vi "SaveImagesFromArray (SubVI).vi"(8 "error in (no error)":errorcluster, 9 "Array of Images":T1[](array[typedef]), 10 "XY Camera Coordinates":dbl[][](array[numeric]), 11 "Path to save collected images":path=path "E:/XYZstage+Camera_CollectedImages/12-17-2016/images") -> (0 "error out":errorcluster)   [LabVIEW 2016]
uses:
  <vilib>/vision/Image Controls.llb/IMAQ Image.ctl
  <vilib>/Utility/file.llb/Write Delimited Spreadsheet (DBL).vi
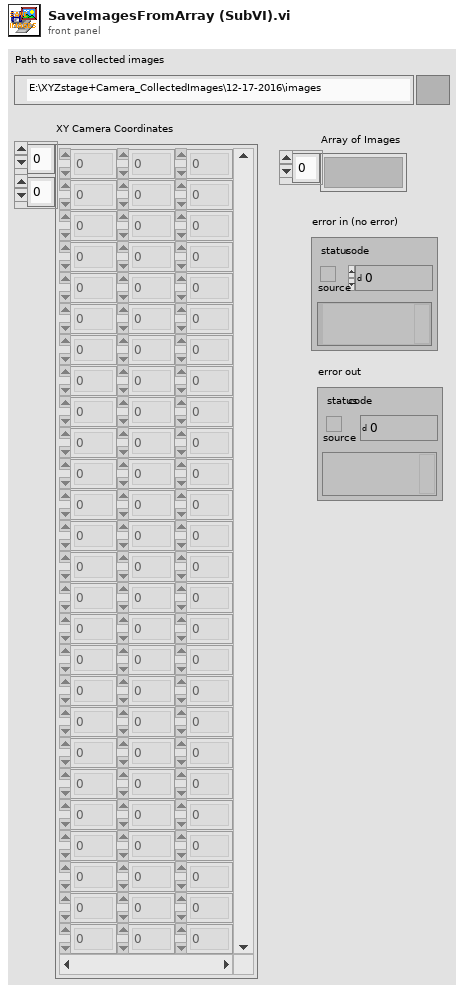
[diagram p1: front panel]
types:
  T1 = typedef "IMAQ Image.ctl" = refnum<image>
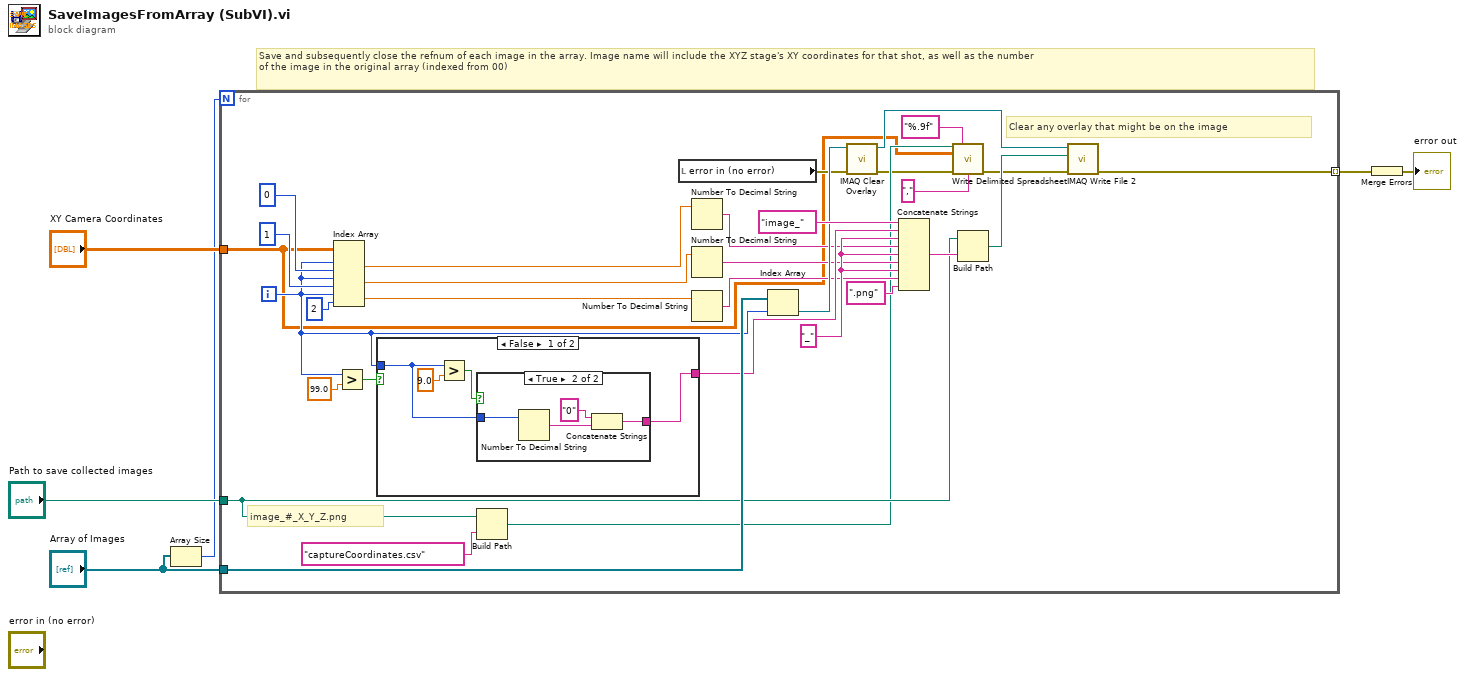
[diagram p0: block diagram]
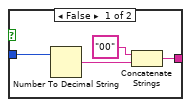
[diagram p2: hidden frame]
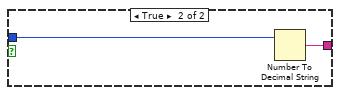
[diagram p3: hidden frame]
diagram:
  # "Save and subsequently close the refnum of each image in the array. Image name will include the XYZ stage's XY coordinates for that shot, as well as the number\nof the image in the original array (indexed from 00)"
  n1 = Array Size(array="Array of Images") -> (size(s)=w3:i32)
  n2 = for {
    N: w3 -> [_]
    tunnel: "Array of Images" -> [w37]
    tunnel: "Path to save collected images" -> [w13]
    tunnel: "XY Camera Coordinates" -> [w11]
    tunnel: [w30] -> w2 mode=indexing
    i -> [w15]
    w22 = "_" ("string")
    # "image_#_X_Y_Z.png"
    # "Clear any overlay that might be on the image"
    n3 = Index Array(array=w11, index (row) #1=w15, index (col) #1=0 ("disabled index (col)"), index (row) #2=w15, index (col) #2=1 ("disabled index (col)"), index (row) #3=w15, index (col) #3=2 ("index (col)")) -> (element #1=w33:dbl, element #2=w31:dbl, element #3=w23:dbl)
    n4 = Greater?(x=w15, y=99.0) -> (0:w17:bool)
    n5 = case shown="False" w17 {
      tunnel: w15 -> [w38 w51]
      tunnel: [w40 w50] -> w21
      frame False {
        n6 = Greater?(x=w38, y=9.0) -> (0:w39:bool)
        n7 = case shown="True" w39 {
          tunnel: [w43 w46] -> w40
          tunnel: w38 -> [w42 w47]
          frame False {
            n8 = Number To Decimal String(number=w42) -> (decimal integer string=w45:string)  [unwired: 1 in]
            n9 = Concatenate Strings("00" ("string"), w45) -> (w43:string)
          }
          frame True {
            n10 = Number To Decimal String(number=w47) -> (decimal integer string=w49:string)  [unwired: 1 in]
            n11 = Concatenate Strings("0" ("string"), w49) -> (w46:string)
          }
        }
      }
      frame True {
        n12 = Number To Decimal String(number=w51) -> (decimal integer string=w50:string)  [unwired: 1 in]
      }
    }
    n13 = Build Path(base path=w13, name or relative path="captureCoordinates.csv") -> (appended path=w12:path)
    n14 = local read "error in (no error)"() -> (w28:errorcluster)
    n15 = Number To Decimal String(number=w33) -> (decimal integer string=w20:string)  [unwired: 1 in]
    n16 = Number To Decimal String(number=w31) -> (decimal integer string=w19:string)  [unwired: 1 in]
    n17 = Number To Decimal String(number=w23) -> (decimal integer string=w18:string)  [unwired: 1 in]
    n18 = Index Array(array=w37, index=w15) -> (element=w29:T1)
    n19 = call "IMAQ Clear Overlay"("error in (no error)"=w28, "Image"=w29) -> ("error out"=w10:errorcluster, "Image Out"=w27:T1)  [unwired: 8 in]
    n20 = Concatenate Strings("image_" ("string"), w21, w22, w20, w22, w19, w22, w18, ".png" ("string")) -> (w36:string)
    n21 = call-poly <vilib>:"Write Delimited Spreadsheet.vi"("file path (dialog if empty)"=w12, "format (%.3f)"="%.9f", "2D data"=w11, "error in (no error)"=w10, "delimiter (\\t)"="," ("delimiter (\\t)")) -> ("error out"=w9:errorcluster)  [unwired: 9 in, 1 out]
    n22 = Build Path(base path=w13, name or relative path=w36) -> (appended path=w26:path)
    n23 = call-poly "IMAQ Write File 2"("error in (no error)"=w9, "File Path"=w26, "Image"=w27) -> ("error out"=w30:errorcluster)  [unwired: 7 in, 1 out]
  }
  n24 = Merge Errors(w2) -> (→"error out":errorcluster)
